vi "ENPH354_A1.vi"() -> ()   [LabVIEW 2020]
uses:
  <vilib>/numeric/Random Number (Range) U64.vi
  <vilib>/numeric/sub_Random U32.vi
panel:
  in  "Q7_BinNum":bool[](array[boolean])
  out "Q7_Decimal number":dbl
  out "Q6_RandNumsPos":dbl[](array[numeric])
  out "Q6_RandNumsNeg":dbl[](array[numeric])
  out "Q5_RandomNumber":dbl
  out "Q5_NumberInRange":string
  out "Q4_Hello 2023 :)":string
  in  "Q4_Hello  2022":string
  out "Q3_NvsSum":dbl[][](array[numeric])
  out "Q2_2DArray":dbl[][](array[numeric])
  out "Q1_RandArray":dbl[](array[numeric])
  out "Q1_RandArrayAvg":dbl
  # "Q1"
  # "Q2"
  # "Q3"
  # "Q4"
  # "Q5"
  # "Q6"
  # "Q7"
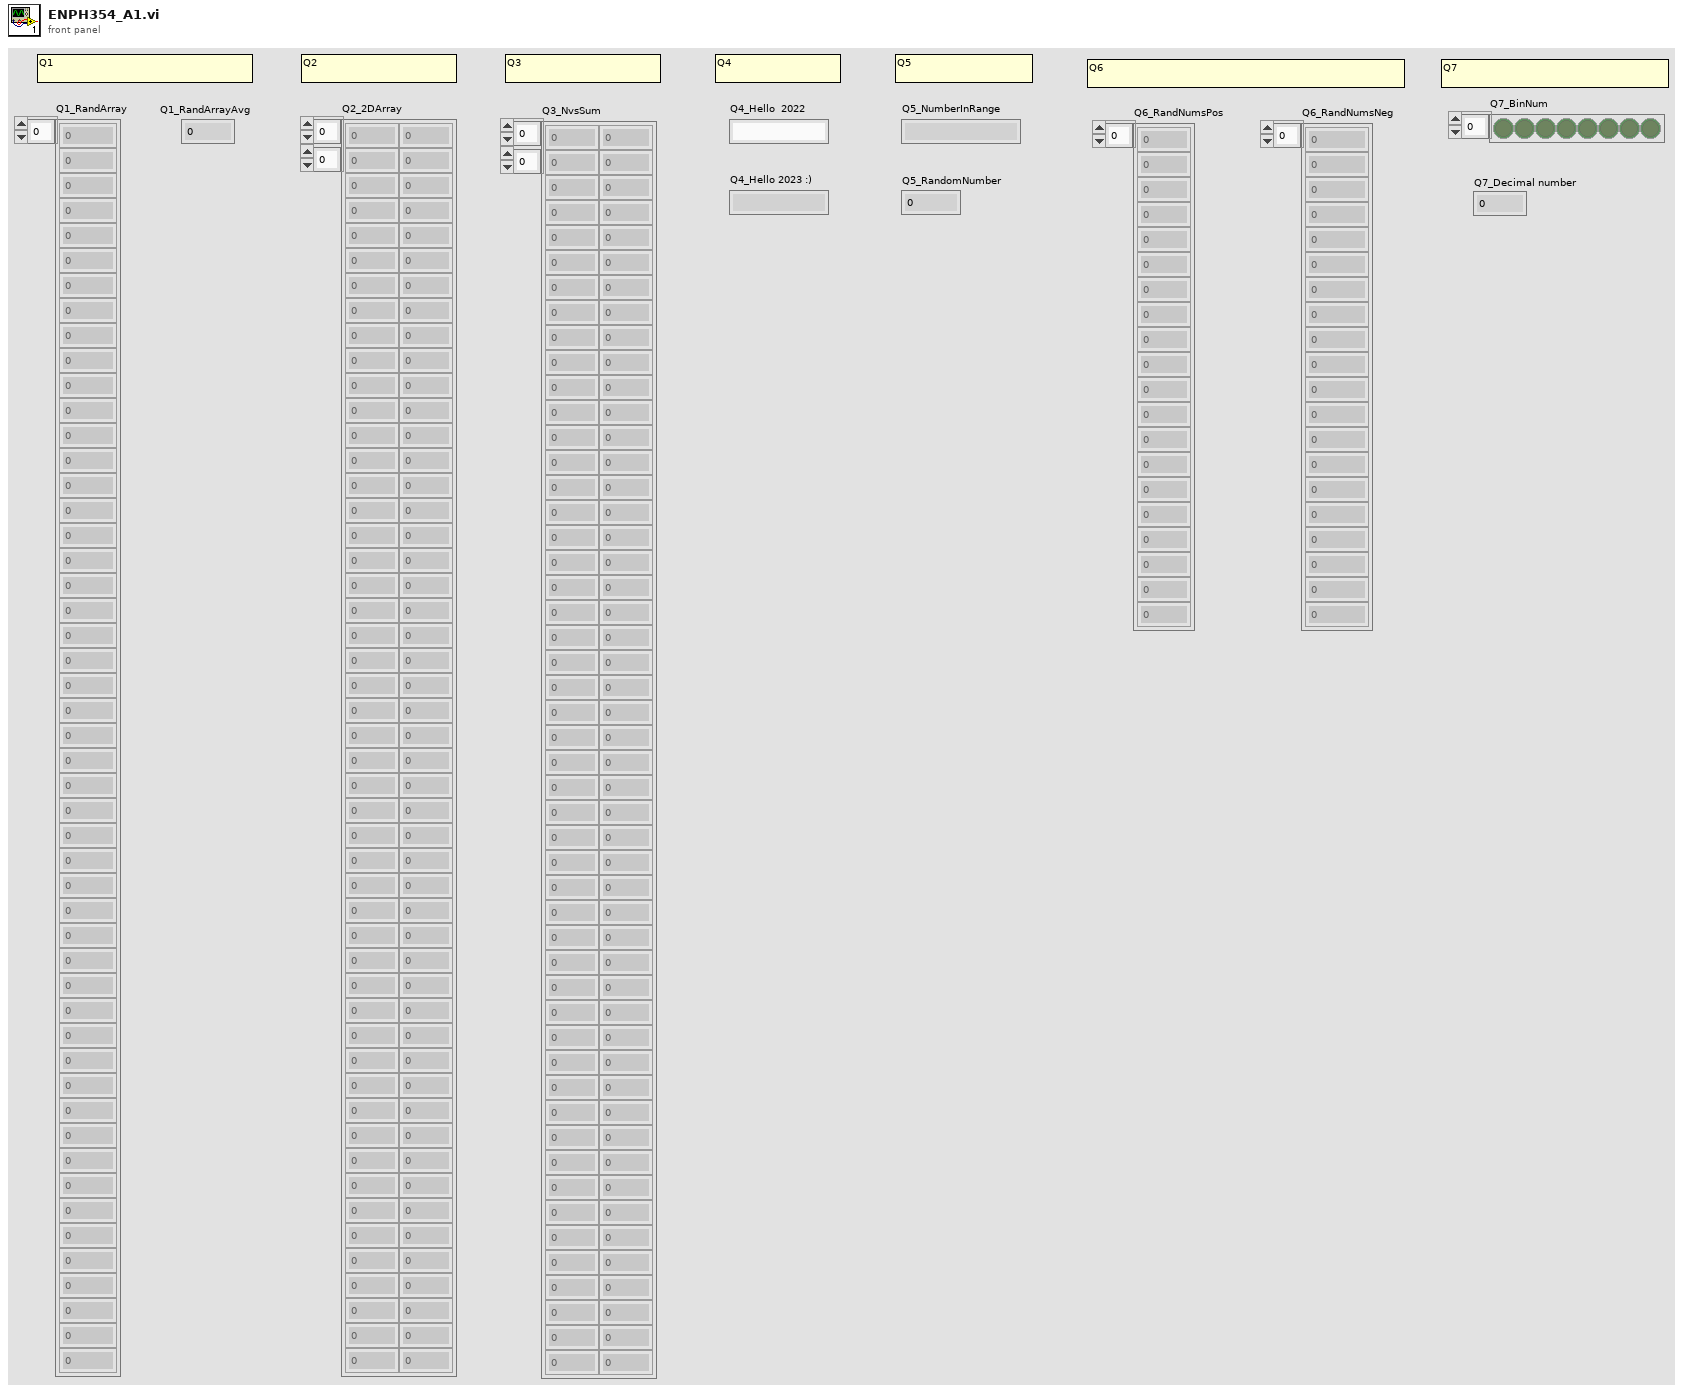
[diagram p1: front panel]
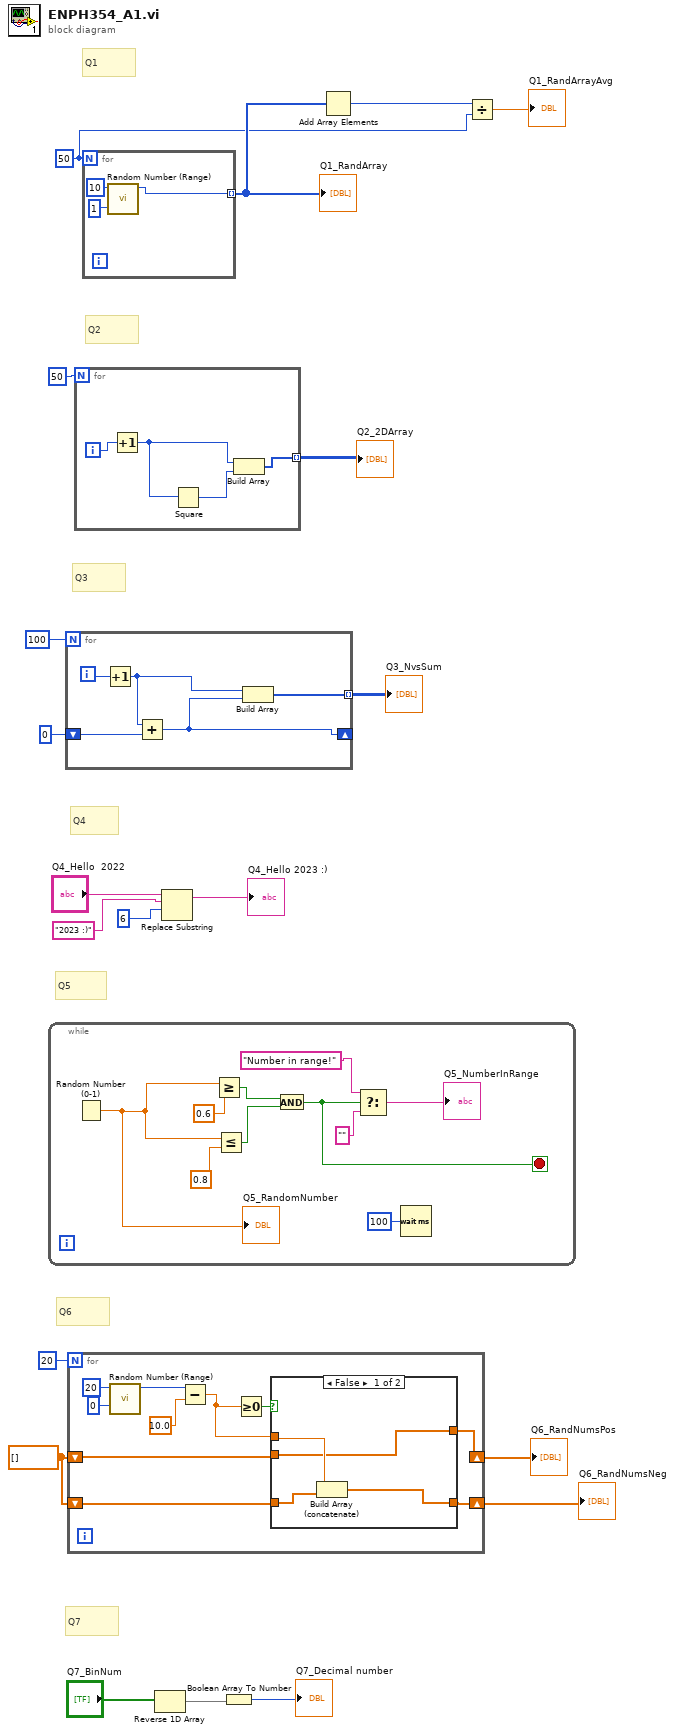
[diagram p0: block diagram]
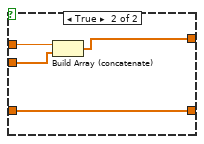
[diagram p2: hidden frame]
diagram:
  w2 = dbl[] []
  w1 = 50
  # "Q7"
  # "Q6"
  # "Q5"
  # "Q4"
  # "Q3"
  # "Q2"
  # "Q1"
  n1 = while {
    stop <- w25 stop-if-true
    n2 = Random Number (0-1)() -> (number: 0 to 1=w22:dbl)
    "Q5_RandomNumber" <- w22
    n3 = Greater Or Equal?(x=w22, y=0.6 ("x")) -> (x >= y?=w29:bool)
    n4 = Less Or Equal?(x=w22, y=0.8) -> (x <= y?=w28:bool)
    n5 = And(x=w29, y=w28) -> (x .and. y?=w25:bool)
    n6 = Select(t="Number in range!", s=w25, f="") -> (s? t:f=→"Q5_NumberInRange":string)
    n7 = Wait (ms)(milliseconds to wait=u32 100) -> ()  [unwired: 1 out]
  }
  n8 = for {
    N: 100 -> [_]
    shift-right: [w33] -> _
    shift-left: 0 -> [w34]
    tunnel: [w32] -> w6 mode=indexing
    i -> [w35]
    n9 = Increment(x=w35) -> (x+1=w31:i32)
    n10 = Add(x=w31, y=w34) -> (x+y=w33:i32)
    n11 = Build Array(w31, w33) -> (w32:i32[])
  }
  "Q3_NvsSum" <- w6
  n12 = for {
    N: 20 -> [_]
    shift-right: [w39] -> w4
    shift-left: w2 -> [w37]
    shift-right: [w38] -> w3
    shift-left: w2 -> [w36]
    n13 = call-poly <vilib>:"Random Number (Range).vi"("lower bound (0)"=u64 0, "upper bound (100)"=u64 20) -> ("number"=w42:u64)  [unwired: 9 in]
    n14 = Subtract(x=w42, y=10.0) -> (x-y=w40:dbl)
    n15 = Greater Or Equal To 0?(x=w40) -> (x >= 0?=w41:bool)
    n16 = case shown="False" w41 {
      tunnel: w40 -> [w49 w53]
      tunnel: w37 -> [w46 w50]
      tunnel: [w46 w52] -> w39
      tunnel: [w48 w51] -> w38
      tunnel: w36 -> [w47 w51]
      frame False {
        n17 = Build Array (concatenate)(w49, w47) -> (w48:dbl[])
      }
      frame True {
        n18 = Build Array (concatenate)(w53, w50) -> (w52:dbl[])
      }
    }
  }
  "Q6_RandNumsPos" <- w4
  "Q6_RandNumsNeg" <- w3
  n19 = for {
    N: 50 -> [_]
    tunnel: [w54] -> w17 mode=indexing
    i -> [w57]
    n20 = Increment(x=w57) -> (x+1=w55:i32)
    n21 = Square(x=w55) -> (x^2=w56:i32)
    n22 = Build Array(w55, w56) -> (w54:i32[])
  }
  "Q2_2DArray" <- w17
  n23 = for {
    N: w1 -> [_]
    tunnel: [w58] -> w16 mode=indexing
    n24 = call-poly <vilib>:"Random Number (Range).vi"("lower bound (0)"=u64 1, "upper bound (100)"=u64 10) -> ("number"=w58:u64)  [unwired: 9 in]
  }
  "Q1_RandArray" <- w16
  n25 = Reverse 1D Array(array="Q7_BinNum") -> (reversed array=w10:bool[])
  n26 = Replace Substring(3:6 ("offset (0)"), 4:"2023 :)", 5:"Q4_Hello  2022") -> (1:→"Q4_Hello 2023 :)":string)  [unwired: 1 in, 1 out]
  n27 = Boolean Array To Number(Boolean array=w10) -> (number=→"Q7_Decimal number":u32)
  n28 = Add Array Elements(numeric array=w16) -> (sum=w20:u64)
  n29 = Divide(x=w20, y=w1) -> (x/y=→"Q1_RandArrayAvg":dbl)
